vi "Get Total Data Size.vi"(8 "error in (no error)":errorcluster {"code" format="Error %.0f"}, 11 "GUI Documentation In":refnum<class "GUI Documentation.lvclass">) -> (0 "error out":errorcluster {"code" format="Error %.0f"}, 2 "Total Data Size (MB)":dbl, 3 "GUI Documentation Out":refnum<class "GUI Documentation.lvclass">)   [LabVIEW 2023, in "VIDoc Parsing.lvlib" / "GUI Documentation.lvclass"]
uses:
  GUI Documentation.lvclass
  GUI Documentation.lvclass/GUI Documentation.ctl
  VIDoc Parsing.lvlib
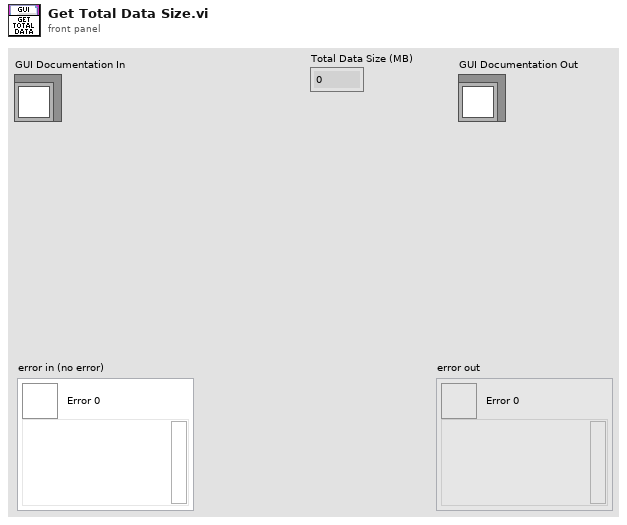
[diagram p1: front panel]
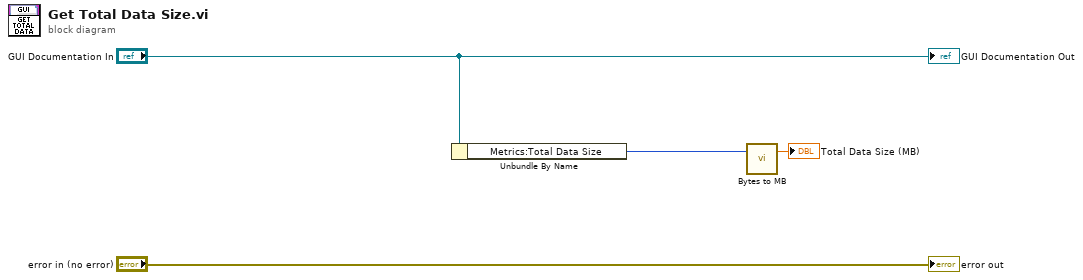
[diagram p0: block diagram]
diagram:
  n1 = Unbundle By Name("GUI Documentation In") -> ("Metrics:Total Data Size"=w1:u32)
  n2 = call "Bytes to MB.vi"("Metrics: Data Size"=w1) -> ("MB"=→"Total Data Size (MB)":dbl)  [unwired: 2 in]
  "error out" <- "error in (no error)"
  "GUI Documentation Out" <- "GUI Documentation In"
